vi "Energy.vi"(9 "data in":u32, 10 "data in valid":bool, 11 "Pulse width":u16) -> (2 "valid":bool, 3 "out":u32)   [LabVIEW 2017]
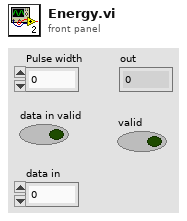
[diagram p1: front panel]
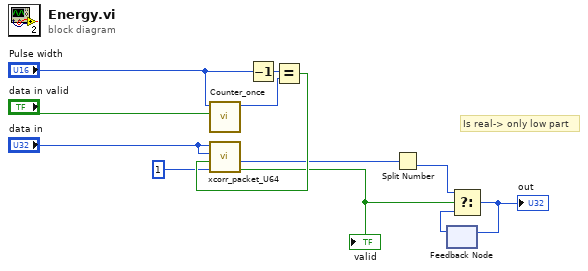
[diagram p0: block diagram]
diagram:
  # "Is real-> only low part"
  n1 = call "Counter_once.vi"("reset"="data in valid", "limit"="Pulse width") -> ("count"=w10:u16)  [unwired: 9 in]
  n2 = Decrement(x="Pulse width") -> (x-1=w9:u16)
  n3 = Equal?(x=w9, y=w10) -> (x = y?=w11:bool)
  n4 = call "xcorr_packet_U64.vi"("x"="data in", "y"="data in", "trigger"=w11, "normalization"=u8 1) -> ("out"=w2:u64, "valid"=w5:bool)  [unwired: 4 in]
  "valid" <- w5
  n5 = Split Number(x=w2) -> (lo(x)=w1:u32)  [unwired: 1 out]
  n6 = feedback #1() -> (w6:u32)  [unwired: 1 in]
  n7 = Select(t=w1, s=w5, f=w6) -> (s? t:f=w4:u32)
  "out" <- w4
  n8 = feedback-in #1(w4) -> ()
